vi "Format CAN Data.vi"(10 "ID ERROR MESSAGE":u32=255 format="%x", 11 "Frame":T1 {"payload" format="%x"; "timestamp" format="%<%.7X\n%x>T"; "type" items=["CAN Data"=0, "CAN Remote"=1, "CAN Bus Error"=2, "CAN 2.0 Data"=8, "CAN FD Data"=16, "CAN FD+BRS Data"=24, "J1939 Data"=192, "Delay"=224, "Log Trigger"=225, "Start Trigger"=226]; "identifier" format="%x"}) -> (1 "Error":bool, 2 "Error Number":u8, 3 "Display":string[](array[string]))   [LabVIEW 2025, in "Workflow DO.lvclass"]
uses:
  Workflow DO.lvclass
  <vilib>/xnet/xnet.llb/XNET Frame CAN.ctl
  <vilib>/xnet/xnet.llb/XNET Frame Type CAN.ctl
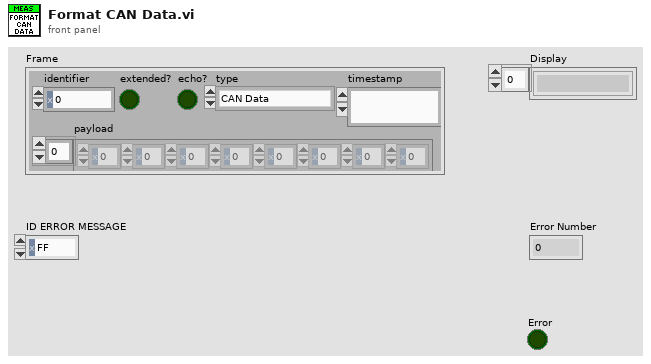
[diagram p1: front panel]
types:
  T1 = typedef "XNET Frame CAN.ctl" = cluster{"timestamp":timestamp, "payload":u8[], "identifier":u32, "type":T2, "extended?":bool, "echo?":bool}
  T2 = typedef "XNET Frame Type CAN.ctl" = u8
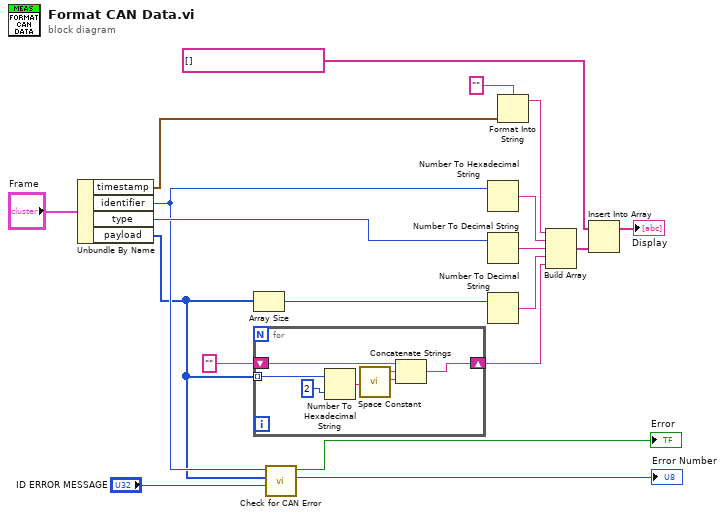
[diagram p0: block diagram]
diagram:
  n1 = Unbundle By Name("Frame") -> ("timestamp"=w8:timestamp, "identifier"=w5:u32, "type"=w7:T2, "payload"=w4:u8[])
  n2 = Array Size(array=w4) -> (size(s)=w15:i32)
  n3 = for {
    tunnel: w4 -> [w25] mode=indexing
    shift-right: [w22] -> w18
    shift-left: "" -> [w21]
    n4 = Number To Hexadecimal String(1:i16 2 ("width (-)"), 2:w25) -> (0:w23:string)
    n5 = call <vilib>:"Space Constant.vi"() -> ("String"=w20:string)
    n6 = Concatenate Strings(w21, w23, w20) -> (w22:string)
  }
  n7 = call "Check for CAN Error.vi"("ID ERROR MESSAGE"="ID ERROR MESSAGE", "payload"=w4, "identifier"=w5) -> ("Error Number"=→"Error Number":u8, "Error"=→"Error":bool)  [unwired: 7 in]
  n8 = Number To Hexadecimal String(2:w5) -> (0:w9:string)  [unwired: 1 in]
  n9 = Number To Decimal String(number=w7) -> (decimal integer string=w14:string)  [unwired: 1 in]
  n10 = Number To Decimal String(number=w15) -> (decimal integer string=w16:string)  [unwired: 1 in]
  n11 = Format Into String(format string="", w8) -> (resulting string=w12:string)  [unwired: 2 in, 1 out]
  n12 = Build Array(w12, w9, w14, w16, w18) -> (w10:string[])
  n13 = Insert Into Array(array=string[] [] ("Display"), new element=w10) -> (→"Display":string[])  [unwired: 1 in]
